vi "SignalGenerator.vi"(9 "stop":bool, 10 "Frequency":i32, 11 "Amplitude":i32=2) -> ()   [LabVIEW 2014]
panel:
  out "error out 2":errorcluster caption="error out"
  in  "error in (no error)":errorcluster
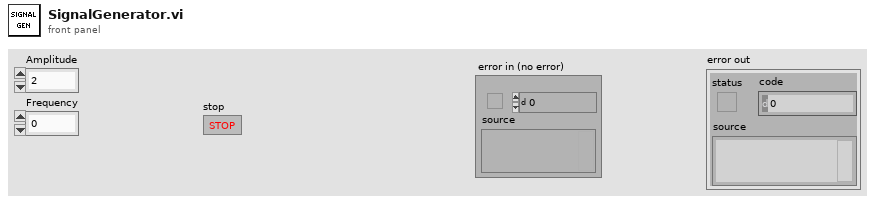
[diagram p1: front panel]
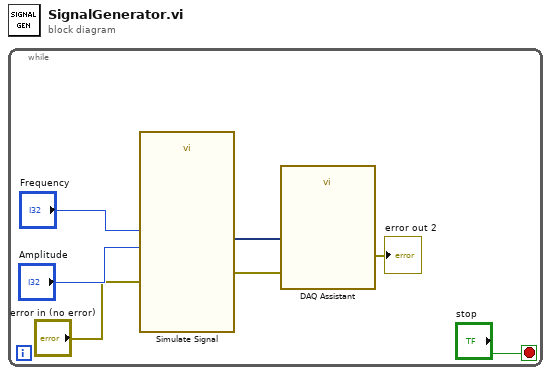
[diagram p0: block diagram]
diagram:
  n1 = while {
    stop <- "stop" stop-if-true
    n2 = call "Simulate Signal"("Frequency"="Frequency", "Amplitude"="Amplitude", "error in (no error)"="error in (no error)") -> ("Sine"=w7:dynamicdata, "error out"=w2:errorcluster)  [unwired: 11 in]
    n3 = call "DAQ Assistant"("data"=w7, "error in"=w2) -> ("error out"=→"error out 2":errorcluster)  [unwired: 15 in, 2 out]
  }
